vi "Read Symbol Attribute.vi"(8 "error in (no error)":errorcluster, 10 "Symbol Name":string, 11 "TwinCAT ADS in":refnum<class "TwinCAT ADS.lvclass">) -> (0 "error out":errorcluster, 2 "Attributes":T1[](array[typedef]), 3 "TwinCAT ADS out":refnum<class "TwinCAT ADS.lvclass">)   [LabVIEW 2018, in "TwinCAT ADS.lvclass"]
uses:
  TwinCAT ADS.lvclass
  Controls/Type Attribute.ctl
  TwinCAT ADS.lvclass/TwinCAT ADS.ctl
  TwinCAT.Ads
  Get From Symbol Map.vi
  Get From Symbol Map Daemon.vi
  Get Symbol Map.vi
  Format String.vi
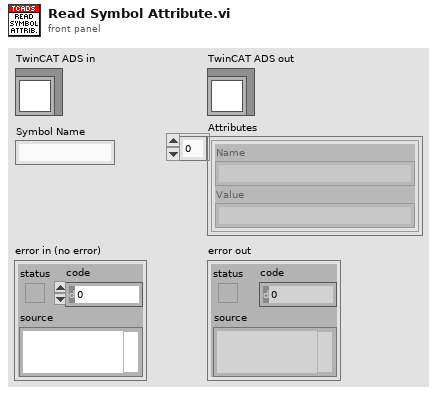
[diagram p1: front panel]
types:
  T1 = typedef "TwinCAT ADS.lvclass/Type Attribute.ctl" = cluster{"Name":string, "Value":string}
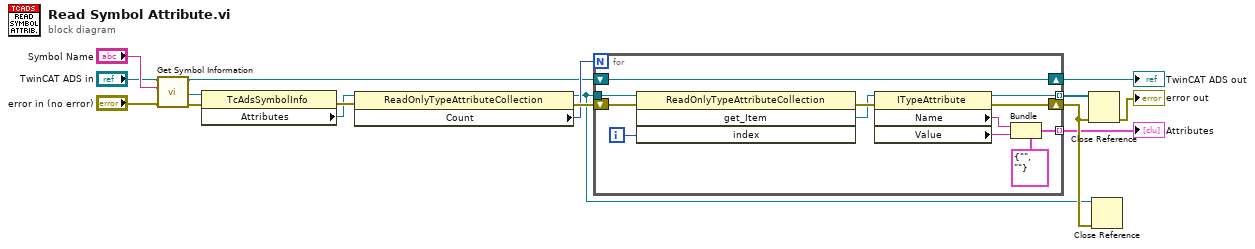
[diagram p0: block diagram]
diagram:
  n1 = call "Get Symbol Information.vi"("error in (no error)"="error in (no error)", "Symbol Name"="Symbol Name", "TwinCAT ADS in"="TwinCAT ADS in") -> ("error out"=w5:errorcluster, ".NET Symbol Information"=w4:refnum<k24>, "TwinCAT ADS out"=w1:refnum<class "TwinCAT ADS.lvclass">)  [unwired: 6 in]
  n2 = property class="TcAdsSymbolInfo"(reference=w4, error in=w5) -> (error out=w16:errorcluster, "Attributes"=w15:refnum<k24>)  [unwired: 1 out]
  n3 = property class="ReadOnlyTypeAttributeCollection"(reference=w15, error in=w16) -> (reference out=w8:refnum<k24>, error out=w14:errorcluster, "Count"=w13:i32)
  n4 = for {
    N: w13 -> [_]
    tunnel: w8 -> [w27]
    shift-right: [w22] -> w9
    shift-left: w14 -> [w28]
    shift-right: [w21] -> w12
    shift-left: w1 -> [w21]
    tunnel: [w18] -> w7 mode=indexing
    tunnel: [w17] -> w11 mode=indexing
    i -> [w20]
    n5 = invoke class="ReadOnlyTypeAttributeCollection" method="get_Item"(reference=w27, error in=w28, "index"=w20) -> (error out=w26:errorcluster, "get_Item"=w23:refnum<k24>)  [unwired: 1 in, 2 out]
    n6 = property class="ITypeAttribute"(reference=w23, error in=w26) -> (reference out=w17:refnum<k24>, error out=w22:errorcluster, "Name"=w25:string, "Value"=w24:string)
    n7 = Bundle(cluster=T1 {"Name"="", "Value"=""} ("Type Attribute"), "Name"=w25, "Value"=w24) -> (w18:T1)
  }
  "TwinCAT ADS out" <- w12
  "Attributes" <- w7
  n8 = Close Reference(reference=w11, error in (no error)=w9) -> (error out=→"error out":errorcluster)
  n9 = Close Reference(reference=w8, error in (no error)=w9) -> ()  [unwired: 1 out]
